vi "Set DataList Tree Property.vi"(7 "file path":path, 8 "error in (no error)":errorcluster, 10 "Group&ChName":cluster{"Group":string, "ChName":string[]}[](array[cluster]), 11 "Tree Ref":refnum<vi>) -> (0 "error out":errorcluster, 3 "Tree Ref":refnum<vi>)   [LabVIEW 2012]
doc: "设置通道列表树形控件属性。"
panel:
  in  "Cluster":cluster{"Index":i32, "Picture Path":path}
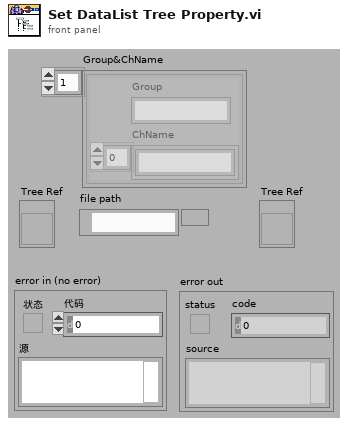
[diagram p1: front panel]
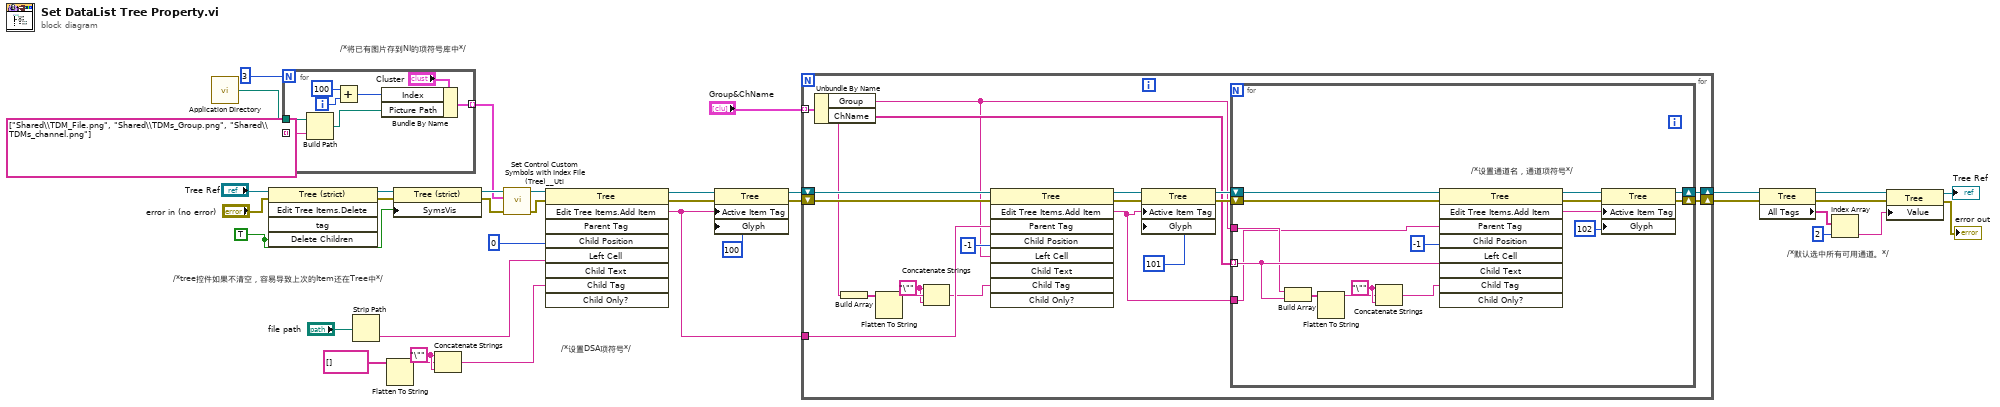
[diagram p0: block diagram]
diagram:
  w9 = "\"" ("string")
  w19 = TRUE ("删除子项？")
  # "/*将已有图片存到NI的项符号库中*/"
  # "/*tree控件如果不清空，容易导致上次的Item还在Tree中*/"
  # "/*默认选中所有可用通道。*/"
  # "/*设置DSA项符号*/"
  n1 = call <vilib>:"Application Directory.vi"() -> ("Application Directory"=w14:path)
  n2 = invoke class="Tree (strict)" method="Edit Tree Items.Delete"(reference="Tree Ref", error in="error in (no error)", "Delete Children"=w19) -> (reference out=w23:refnum<vi>, error out=w22:errorcluster)  [unwired: 2 in, 3 out]
  n3 = for {
    N: 3 -> [_]
    tunnel: [w41] -> w20 mode=indexing
    tunnel: w14 -> [w40]
    tunnel: string[] ["Shared\\TDM_File.png", "Shared\\TDMs_Group.png", "Shared\\TDMs_channel.png"] -> [w39] mode=indexing
    i -> [w44]
    n4 = Build Path(base path=w40, name or relative path=w39) -> (appended path=w37:path)
    n5 = Add(x=100, y=w44) -> (x+y=w38:i32)
    n6 = Bundle By Name(cluster="Cluster", "Index"=w38, "Picture Path"=w37) -> (w41:cluster{"Index":i32, "Picture Path":path})
  }
  n7 = Strip Path(path="file path") -> (name=w6:string)  [unwired: 1 out]
  n8 = Flatten To String(anything=string[] [] ("appended array")) -> (data string=w8:string)  [unwired: 3 in, 2 out]
  n9 = property class="Tree (strict)"(reference=w23, error in=w22, "SymsVis"=w19) -> (reference out=w21:refnum<vi>, error out=w18:errorcluster)
  n10 = Concatenate Strings(w9, w8, w9) -> (w5:string)
  n11 = call "Set Control Custom Symbols with Index File (Tree)__Uti.vi"("error in (no error)"=w18, "custom symbol files with indice"=w20, "tree in"=w21) -> ("error out"=w34:errorcluster, "tree out"=w35:refnum<vi>)  [unwired: 7 in]
  n12 = invoke class="Tree" method="Edit Tree Items.Add Item"(reference=w35, error in=w34, "Child Position"=0 ("子项位置"), "Left Cell"=w6, "Child Tag"=w5) -> (reference out=w32:refnum<vi>, error out=w31:errorcluster, "Edit Tree Items:Add Item"=w4:string)  [unwired: 4 in, 6 out]
  n13 = property class="Tree"(reference=w32, error in=w31, "Active Item Tag"=w4, "Glyph"=100 ("活动项:符号索引")) -> (reference out=w30:refnum<vi>, error out=w29:errorcluster)
  n14 = for {
    tunnel: "Group&ChName" -> [w61] mode=indexing
    tunnel: w4 -> [w51]
    shift-right: [w62] -> w26
    shift-left: w30 -> [w56]
    shift-right: [w63] -> w27
    shift-left: w29 -> [w54]
    w48 = "\"" ("string")
    n15 = Unbundle By Name(w61) -> ("Group"=w46:string, "ChName"=w52:string[])
    n16 = Build Array(w46) -> (w50:string[])
    n17 = Flatten To String(anything=w50) -> (data string=w49:string)  [unwired: 3 in, 2 out]
    n18 = Concatenate Strings(w48, w49, w48) -> (w47:string)
    n19 = invoke class="Tree" method="Edit Tree Items.Add Item"(reference=w56, error in=w54, "Parent Tag"=w51, "Child Position"=-1 ("子项位置"), "Left Cell"=w46, "Child Tag"=w47) -> (reference out=w59:refnum<vi>, error out=w60:errorcluster, "Edit Tree Items:Add Item"=w45:string)  [unwired: 3 in, 6 out]
    n20 = property class="Tree"(reference=w59, error in=w60, "Active Item Tag"=w45, "Glyph"=101 ("活动项:符号索引")) -> (reference out=w55:refnum<vi>, error out=w53:errorcluster)
    n21 = for {
      tunnel: w46 -> [w65]
      shift-right: [w71] -> w63
      shift-left: w53 -> [w77]
      shift-right: [w72] -> w62
      shift-left: w55 -> [w79]
      tunnel: w52 -> [w67] mode=indexing
      tunnel: w45 -> [w64]
      w69 = "\"" ("string")
      # "/*设置通道名，通道项符号*/"
      n22 = Build Array(w65, w67) -> (w70:string[])
      n23 = Flatten To String(anything=w70) -> (data string=w68:string)  [unwired: 3 in, 2 out]
      n24 = Concatenate Strings(w69, w68, w69) -> (w66:string)
      n25 = invoke class="Tree" method="Edit Tree Items.Add Item"(reference=w79, error in=w77, "Parent Tag"=w64, "Child Position"=-1 ("子项位置"), "Left Cell"=w67, "Child Tag"=w66) -> (reference out=w76:refnum<vi>, error out=w75:errorcluster, "Edit Tree Items:Add Item"=w73:string)  [unwired: 3 in, 6 out]
      n26 = property class="Tree"(reference=w76, error in=w75, "Active Item Tag"=w73, "Glyph"=102 ("活动项:符号索引")) -> (reference out=w72:refnum<vi>, error out=w71:errorcluster)
    }
  }
  n27 = property class="Tree"(reference=w26, error in=w27) -> (reference out=w28:refnum<vi>, error out=w24:errorcluster, "All Tags"=w3:string[])
  n28 = Index Array(array=w3, index=2 ("索引")) -> (element=w2:string)
  n29 = property class="Tree"(reference=w28, error in=w24, "Value"=w2) -> (reference out=→"Tree Ref":refnum<vi>, error out=→"error out":errorcluster)
